vi "sv_Edge Detection (1 Tach) with IC.vi"(5 "reset? (True)":bool=TRUE, 6 "dt":dbl=11025.0, 7 "slope (Rising)":u16(ring) items=["Rising", "Falling"], 8 "initial conditions":cluster{"x[n]":dbl[], "size":dbl}, 9 "pulse width (2)":i32=2, 10 "threshold (0.0)":dbl format="%.2f", 11 "x[n]":dbl[](array[numeric]) format="%.2f") -> (0 "final conditions":cluster{"x[n]":dbl[], "size":dbl}, 3 "pulse positions [s]":dbl[](array[numeric]) format="%.2f")   [LabVIEW 2017, in "SoundVib_TachProcess.lvlib"]
doc: "Detects the edges in the tachometer pulses contained in <B>x[n]</B> that cross <B>threshold</B>. Perform edge detection to determine the tachometer pulse position. The VI recognizes the points where the signal crosses <B>threshold</B> and <B>x[n]</B> as edges. The VI returns the locations of the detected edges in <B>pulse positions [s]</B>."
uses:
  <vilib>/addons/Sound and Vibration/Order Analysis/Tach Process/SoundVib_TachProcess.lvlib
  <vilib>/Analysis/8numeric.llb/Threshold Detector.vi
panel:
  # "Edge Detection (1 Tach)"
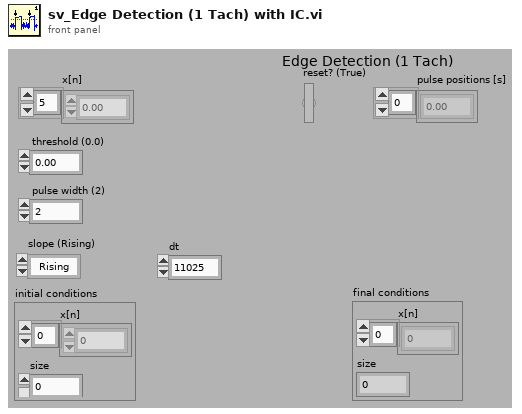
[diagram p1: front panel]
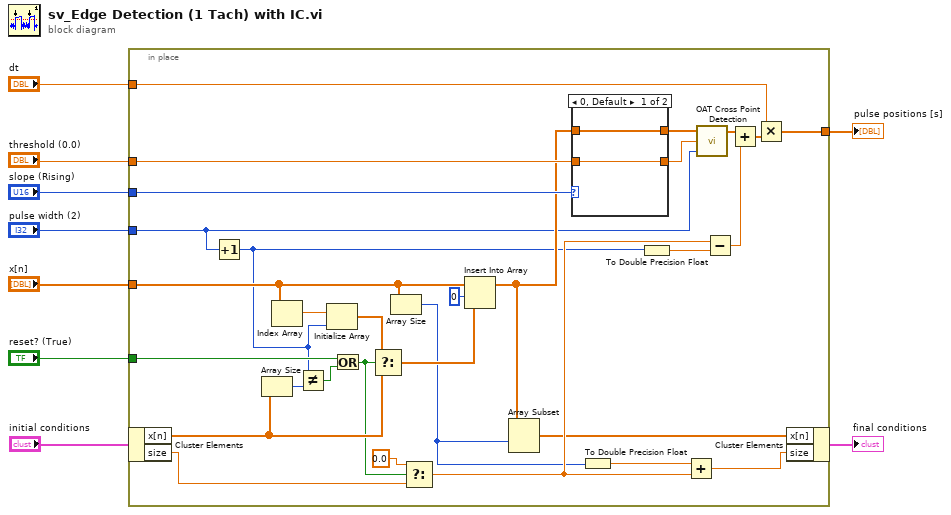
[diagram p0: block diagram]
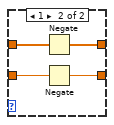
[diagram p2: hidden frame]
diagram:
  n1 = in-place {
    in-place-border: "slope (Rising)" -> [w39]
    in-place-border: "threshold (0.0)" -> [w37]
    in-place-border: [w35] -> w7
    in-place-border: "x[n]" -> [w34]
    in-place-border: "pulse width (2)" -> [w30]
    in-place-border: "dt" -> [w27]
    in-place-border: "reset? (True)" -> [w26]
    n2 = in-place-cluster #1("initial conditions") -> ("x[n]"=w25:dbl[], "size"=w10:dbl)
    n3 = Increment(x=w30) -> (x+1=w13:i32)
    n4 = Array Size(array=w25) -> (size(s)=w22:i32)
    n5 = Index Array(array=w34) -> (element=w23:dbl)  [unwired: 1 in]
    n6 = Not Equal?(x=w13, y=w22) -> (x != y?=w21:bool)
    n7 = Initialize Array(w23, w13) -> (w18:dbl[])
    n8 = Or(x=w26, y=w21) -> (x .or. y?=w17:bool)
    n9 = Select(t=w18, s=w17, f=w25) -> (s? t:f=w20:dbl[])
    n10 = Array Size(array=w34) -> (size(s)=w15:i32)
    n11 = Select(t=0.0, s=w17, f=w10) -> (s? t:f=w31:dbl)
    n12 = Insert Into Array(array=w34, index=0 ("Index"), new element=w20) -> (w33:dbl[])
    n13 = Array Subset(array=w33, index=w15) -> (w24:dbl[])  [unwired: 1 in]
    n14 = case shown="0, Default" w39 {
      tunnel: w37 -> [w40 w43]
      tunnel: w33 -> [w41 w45]
      tunnel: [w41 w44] -> w36
      tunnel: [w40 w42] -> w38
      frame 0, Default {
      }
      frame 1 {
        n15 = Negate(x=w45) -> (-x=w44:dbl[])
        n16 = Negate(x=w43) -> (-x=w42:dbl)
      }
    }
    n17 = To Double Precision Float(number=w15) -> (double precision float=w14:dbl)
    n18 = To Double Precision Float(number=w13) -> (double precision float=w12:dbl)
    n19 = Add(x=w14, y=w31) -> (x+y=w11:dbl)
    n20 = call <vilib>:"OAT Cross Point Detection.vi"("pulse width (2)"=w30, "threshold (0)"=w38, "data in"=w36) -> ("edge position"=w32:dbl[])  [unwired: 1 in]
    n21 = Subtract(x=w31, y=w12) -> (x-y=w29:dbl)
    n22 = Add(x=w32, y=w29) -> (x+y=w28:dbl[])
    n23 = Multiply(x=w27, y=w28) -> (x*y=w35:dbl[])
    n24 = in-place-cluster #1("x[n]"=w24, "size"=w11) -> (→"final conditions":cluster{"x[n]":dbl[], "size":dbl})
  }
  "pulse positions [s]" <- w7
